vi "MeasureInLoop.vi"() -> ()   [LabVIEW 2022 SP3]
uses:
  Anemometry Sub Vis/Controls/MeasureInLoop.ctl
  Anemometry Sub Vis/File/Setup_Filetype.ctl
  Anemometry Sub Vis/Controls/Post_Process.ctl
  Anemometry Sub Vis/Controls/Save_Data.ctl
  Anemometry Sub Vis/Controls/Setup.ctl
  Anemometry Sub Vis/Globals/Meas_global.vi
  Anemometry Sub Vis/Globals/Trav_pos_global.vi
  Anemometry Sub Vis/Globals/Preference_global.vi
panel:
  out "size(s)":i32
  in  "Tab Control":enum32{"Setup", "MeasGraph2", "Debug"}(tab)
  in  "Setup:":string(combo)="Current_Setup.xls"
  in  "File by:":enum16{"Day", "Week", "Month"}(ring)=enum."Week"
  in  "Measure (seconds)":dbl=60.0
  in  "Wait (minutes)":dbl=15.0
  out "MeasurementsTaken:":i32
  out "XY Graph":cluster{"X array":dbl[], "Y array":dbl[]}[](graph)
  out "CurrentFilename":string
  out "Task":T1=enum."Initialise"
  in  "Stop Button":bool
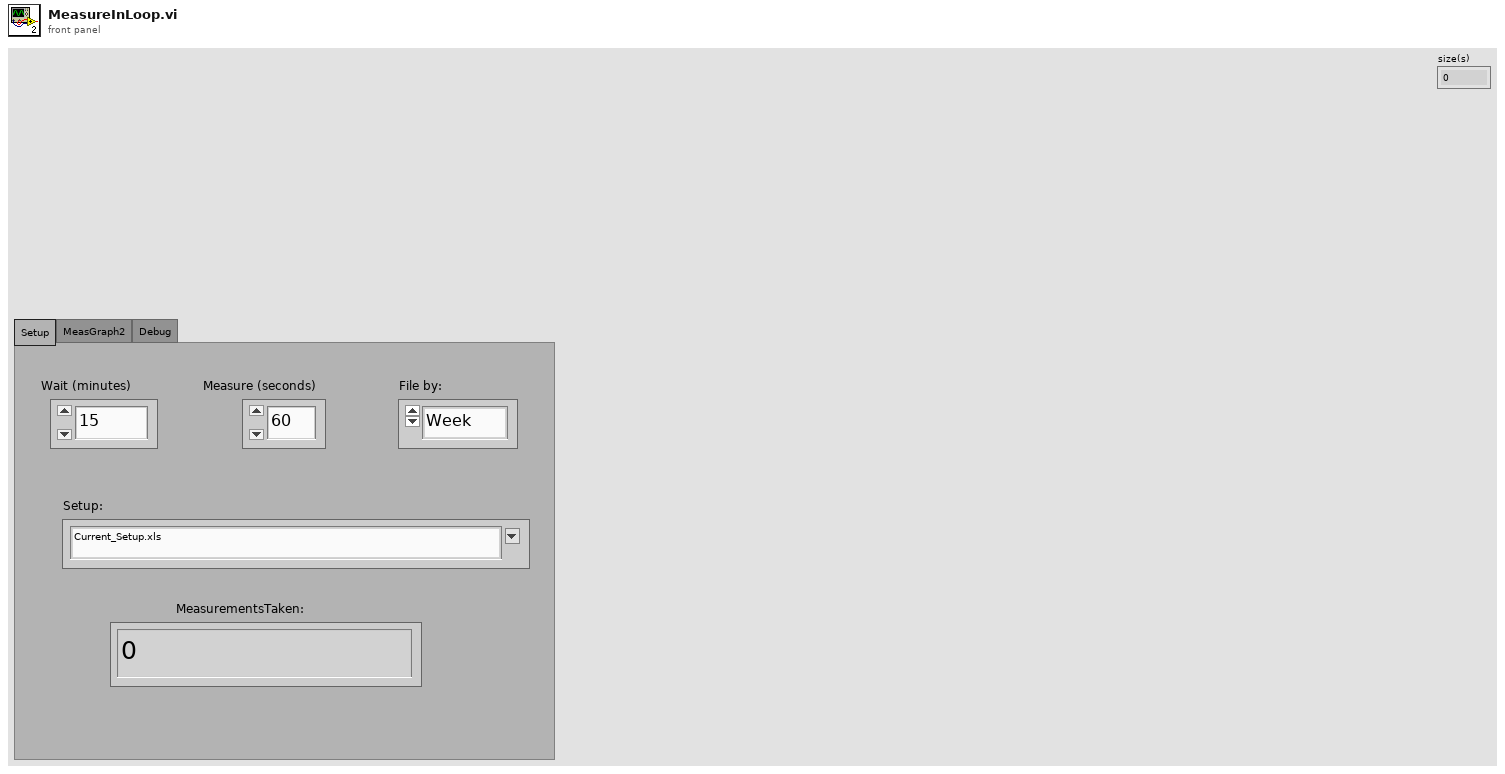
[diagram p1: front panel]
types:
  T1 = typedef "MeasureInLoop.ctl" = enum16{"RunHub", "Initialise", "WaitForServer", "Take Measurement", "Start Waiting", "End"}
  T2 = typedef "Setup.ctl" = enum16{"Run Program", "Show Setup", "Save Current Setup", "Setup Front Panel"}
  T3 = typedef "Save_Data.ctl" = enum16{"Save No Data", "Save Data"}
  T4 = typedef "Post_Process.ctl" = enum16{"Take New Data", "Post Process Raw Data File"}
  T5 = typedef "Setup_Filetype.ctl" = enum16{"Measurement Setups", "Calibration Setups", "General", "Results File Plotter Setups", "Speed Calib Tweaks"}
  T6 = typedef "Server_Comms.ctl" = enum16{"Do Not Link To Server", "Server Link Healthy"}
  T7 = typedef "Traverse_cluster.ctl" = cluster{"Start X":sgl, "Start Y":sgl, "Start Z":sgl, "End X":sgl, "End Y":sgl, "End Z":sgl, "nPoints":i32, "Spacing":T8, "Filename":path, "Tunnel Speed":dbl, "Averaging time (mins)":dbl, "Extra Commands":string, "Carrier_1 Q (l/min)":dbl, "Carrier_2 Q (l/min)":dbl, "Trace Gas Concentration (%)":dbl, "Specific Arguments":string, "Comments":string, "Row No":i32, "Row Type Selector":T9, "EstCompl":string, "Row Duration (mins)":dbl, "nValidPoints":i32, "Meas Setup File":string}
  T8 = typedef "Spacing.ctl" = enum16{"Linear", "Log", "Gauss", "Specified", "N/A"}
  T9 = typedef "Multi_run_mode.ctl" = enum16{"Move Traverse Only", "Set Tunnel Speed Only", "Set Source Only", "Set Measurement Conditions", "Single Measurement", "Vertical Profile", "Lateral Profile", "Longitudinal Profile", "Multi-Axis Profile", "Explore Volume", "Auto Calibrate", "Meas Fast FID Bkgnd", "Check Beam Power", "Scanning Valve Measurement", "Run VI Named:", "Set ADAM Ch", "Wait (minutes)", "Send Message", "Synchronize With:", "Fall Back to this Row", "Turn Off Row Repeating", "Traverse 3D Volume", "Blank Row", "Jump to Fall Back Row"}
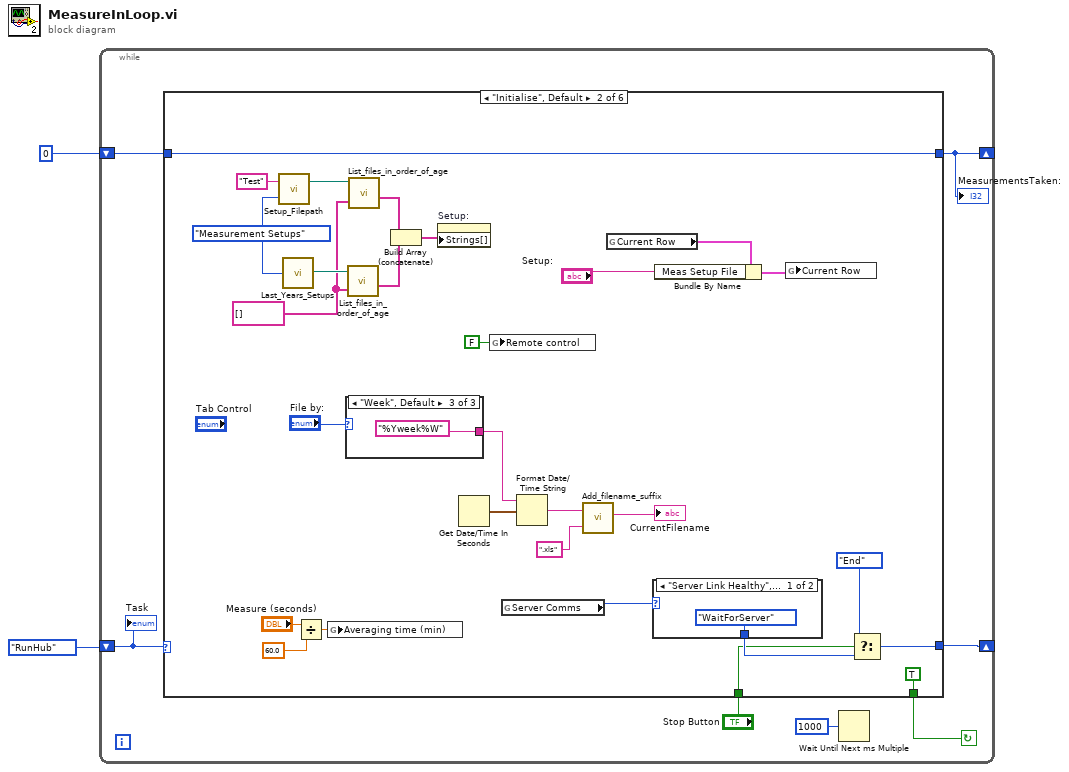
[diagram p0: block diagram]
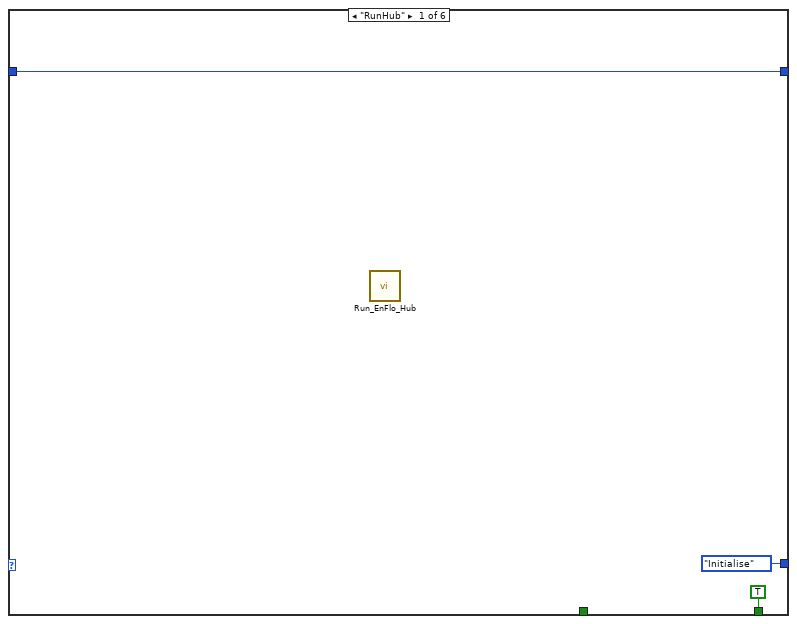
[diagram p2: hidden frame]
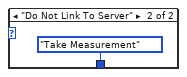
[diagram p3: hidden frame]
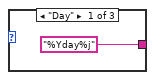
[diagram p4: hidden frame]
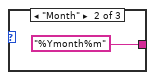
[diagram p5: hidden frame]
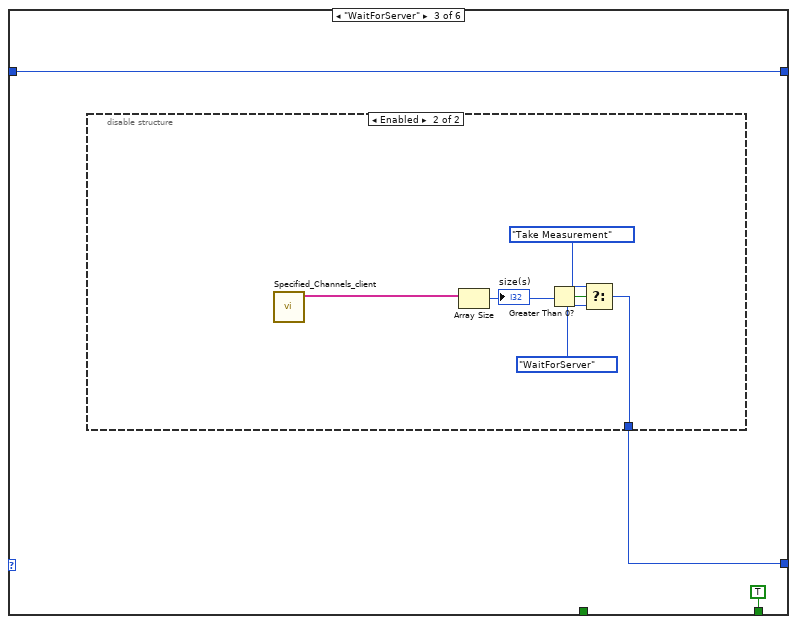
[diagram p6: hidden frame]
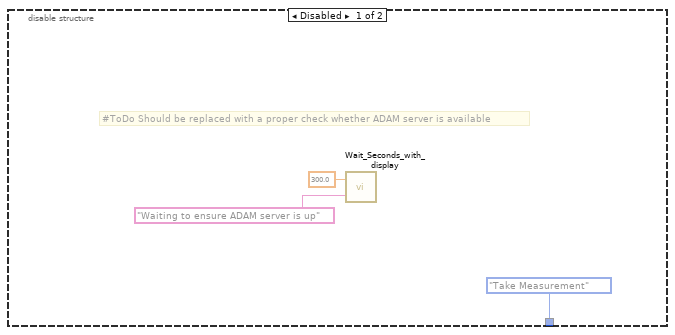
[diagram p7: hidden frame]
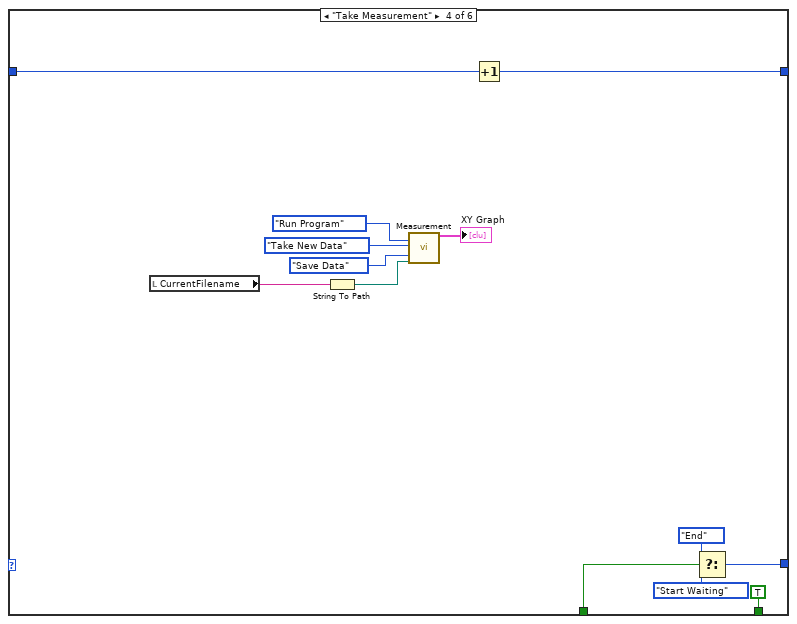
[diagram p8: hidden frame]
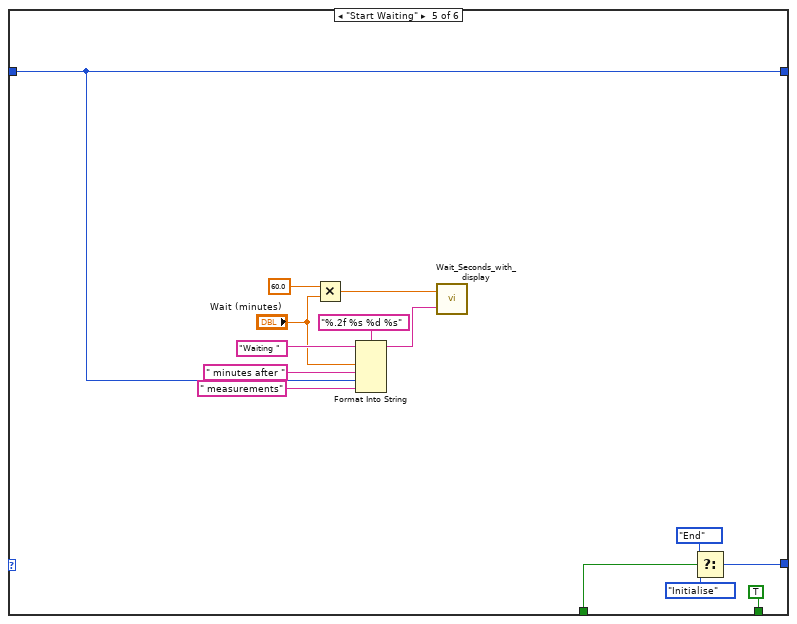
[diagram p9: hidden frame]
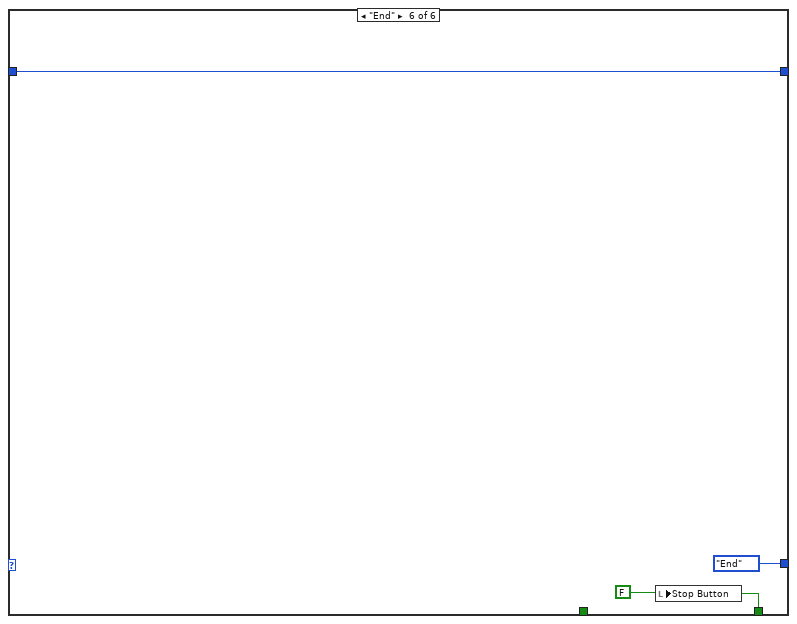
[diagram p10: hidden frame]
diagram:
  n1 = while {
    shift-right: [w9] -> _
    shift-left: MeasureInLoop."RunHub" ("Task") -> [w7]
    shift-right: [w3] -> _
    shift-left: 0 -> [w4]
    stop <- w8 continue-if-true
    n2 = case shown="\"Initialise\", Default" w7 {
      tunnel: [MeasureInLoop."Initialise" ("Task") w17 w47 w63 w74 MeasureInLoop."End" ("Task")] -> w9
      tunnel: [TRUE ("Stop Button") TRUE ("Stop Button") TRUE ("Stop Button") TRUE ("Stop Button") TRUE ("Stop Button") w86] -> w8
      tunnel: "Stop Button" -> [_ w15 _ w60 w72 _]
      tunnel: [w10 w13 w46 w58 w71 w85] -> w3
      tunnel: w4 -> [w10 w13 w46 w59 w71 w85]
      frame "RunHub" {
        n3 = call "Run_EnFlo_Hub.vi"() -> ()  [unwired: 1 in, 7 out]
      }
      frame "Initialise", Default {
        w30 = Setup_Filetype."Measurement Setups" ("Setup File Type")
        w25 = string[] [] ("file names")
        n4 = call "Setup_Filepath.vi"("Setup File Type"=w30, "Filename in"="Test") -> ("Directory"=w29:path)  [unwired: 1 out]
        n5 = call "Last_Years_Setups.vi"("Setup File Type"=w30) -> ("Directory"=w31:path)
        n6 = Divide(x="Measure (seconds)", y=60.0 ("x")) -> (x/y=w32:dbl)
        n7 = global write "Meas_global.vi" "Averaging time (min)"(w32) -> ()
        n8 = case shown="\"Week\", Default" "File by:" {
          tunnel: ["%Yday%j" ("FilenameFormatter") "%Ymonth%m" ("FilenameFormatter") "%Yweek%W" ("FilenameFormatter")] -> w38
          frame "Day" {
          }
          frame "Month" {
          }
          frame "Week", Default {
          }
        }
        n9 = call "List_files_in_order_of_age.vi"("Files to Hide"=w25, "Folder"=w31) -> ("file names"=w27:string[])  [unwired: 9 in]
        n10 = call "List_files_in_order_of_age.vi"("Files to Hide"=w25, "Folder"=w29) -> ("file names"=w28:string[])  [unwired: 9 in]
        n11 = Build Array (concatenate)(w28, w27) -> (w24:string[])
        n12 = property on="Setup:" class="CmbBox"("Strings[]"=w24) -> ()  [unwired: 2 in, 2 out]
        n13 = Get Date/Time In Seconds() -> (seconds since 1Jan1904=w40:timestamp)
        n14 = global write "Meas_global.vi" "Remote control"(FALSE ("Remote control")) -> ()
        n15 = global read "Preference_global.vi" "Server Comms"() -> (w14:T6)
        n16 = Format Date/Time String(time format string (%c)=w38, seconds (now)=w40) -> (date/time string=w37:string)  [unwired: 1 in]
        n17 = call "Add_filename_suffix.vi"("Filename"=w37, "Suffix to add"=".xls") -> ("Filename out"=→"CurrentFilename":string)  [unwired: 3 out]
        n18 = global read "Trav_pos_global.vi" "Current Row"() -> (w22:T7)
        n19 = case shown="\"Server Link Healthy\", Default" w14 {
          tunnel: [MeasureInLoop."WaitForServer" ("Task") MeasureInLoop."Take Measurement" ("Task")] -> w18
          frame "Server Link Healthy", Default {
          }
          frame "Do Not Link To Server" {
          }
        }
        n20 = Bundle By Name(cluster=w22, "Meas Setup File"="Setup:") -> (w21:T7)
        n21 = global write "Trav_pos_global.vi" "Current Row"(w21) -> ()
        n22 = Select(t=MeasureInLoop."End" ("Task"), s=w15, f=w18) -> (s? t:f=w17:T1)
      }
      frame "WaitForServer" {
        n23 = disable-structure shown="Enabled" {
          disable-tunnel: [MeasureInLoop."Take Measurement" ("Task") w53] -> w47
          frame Disabled {
            # "#ToDo Should be replaced with a proper check whether ADAM server is available"
            n24 = call "Wait_Seconds_with_display.vi"("Message"="Waiting to ensure ADAM server is up", "Seconds to wait"=300.0) -> ()  [unwired: 1 in, 1 out]
          }
          frame Enabled {
            n25 = call "Specified_Channels_client.vi"() -> ("All Active Ch Names"=w57:string[])  [unwired: 7 in, 4 out]
            n26 = Array Size(array=w57) -> (size(s)=w56:i32)
            "size(s)" <- w56
            n27 = Greater Than 0?(x=w56) -> (x > 0?=w55:bool)
            n28 = Select(t=MeasureInLoop."Take Measurement" ("Task"), s=w55, f=MeasureInLoop."WaitForServer" ("Task")) -> (s? t:f=w53:T1)
          }
        }
      }
      frame "Take Measurement" {
        n29 = local read "CurrentFilename"() -> (w65:string)
        n30 = String To Path(string=w65) -> (path=w70:path)
        n31 = call "Measurement.vi"("setup"=Setup."Run Program", "Post Process"=Post_Process."Take New Data", "File"=Save_Data."Save Data", "Results file"=w70) -> ("2nd plot"=→"XY Graph":cluster{"X array":dbl[], "Y array":dbl[]}[])  [unwired: 2 in, 13 out]
        n32 = Increment(x=w59) -> (x+1=w58:i32)
        n33 = Select(t=MeasureInLoop."End" ("Task"), s=w60, f=MeasureInLoop."Start Waiting" ("Task")) -> (s? t:f=w63:T1)
      }
      frame "Start Waiting" {
        n34 = Multiply(x=60.0 ("value"), y="Wait (minutes)") -> (x*y=w84:dbl)
        n35 = Format Into String(format string="%.2f %s %d %s", initial string="Waiting " ("Message"), "Wait (minutes)", " minutes after " ("Message"), w71, " measurements" ("Message")) -> (resulting string=w81:string)  [unwired: 1 in, 1 out]
        n36 = call "Wait_Seconds_with_display.vi"("Message"=w81, "Seconds to wait"=w84) -> ()  [unwired: 1 in, 1 out]
        n37 = Select(t=MeasureInLoop."End" ("Task"), s=w72, f=MeasureInLoop."Initialise" ("Task")) -> (s? t:f=w74:T1)
      }
      frame "End" {
        w86 = FALSE ("Stop Button")
        n38 = local write "Stop Button"(w86) -> ()
      }
    }
    "MeasurementsTaken:" <- w3
    n39 = Wait Until Next ms Multiple(millisecond multiple=u32 1000) -> ()  [unwired: 1 out]
    "Task" <- w7
  }
